vi "Begin.vi"(8 "error in":errorcluster) -> (0 "error out":errorcluster)   [LabVIEW 2020]
doc: "Called before other user functions, this VI is expected to open initial I/O refnums, load in file data, and do all program initialization. Notice that the <B>error out</B> terminal is simply used for data flow. Wiring it to other structures or subVIs ensures that this VI runs first."
uses:
  <vilib>/Rock Robotics/WPI/DriverStation/WPI_DriverStationRobotMode2.ctl
  <vilib>/Rock Robotics/WPI/Joystick/WPI_JoystickDeviceEnum.ctl
  <vilib>/Rock Robotics/WPI/Solenoid/WPI_SolenoidChannel.ctl
  <vilib>/Rock Robotics/SystemInterfaces/DIO/FPGA_DIOPWMChannel.ctl
  <vilib>/Rock Robotics/SystemInterfaces/DIO/FPGA_DIOChannel.ctl
  <vilib>/Rock Robotics/SystemInterfaces/AI/FPGA_AIChannel.ctl
  Robot Global Data.vi
  <vilib>/Rock Robotics/WPI/Solenoid/WPI_SolenoidOpenDouble.vi
  <vilib>/Rock Robotics/WPI/MotorControl/WPI_MotorControlOpen SPARK.vi
  <vilib>/Rock Robotics/WPI/Accelerometer/InternalAccelerometer/WPI_AccelerometerInternalOpen.vi
  <vilib>/Rock Robotics/WPI/SafetyOutput/WPI_SafetyOutputConfigMenu.ctl
  <vilib>/Rock Robotics/Network Tables/NT Write String Array.vi
  <vilib>/Rock Robotics/SystemInterfaces/AI/FPGA_AIGyroChannel.ctl
  <vilib>/Rock Robotics/SystemInterfaces/DIO/FPGA_DIORelayChannel.ctl
  <vilib>/Rock Robotics/WPI/Ultrasonic/WPI_SonarMB1010AnalogRefNum Registry Set.vi
  <vilib>/Rock Robotics/WPI/Ultrasonic/WPI_SonarMB1010AnalogOpen.vi
  <vilib>/Rock Robotics/WPI/Gyro/WPI_GyroAnalogOpen.vi
  <vilib>/Rock Robotics/WPI/RobotDrive/WPI_RobotDriveOpen2MotorWithVictorSPX.vi
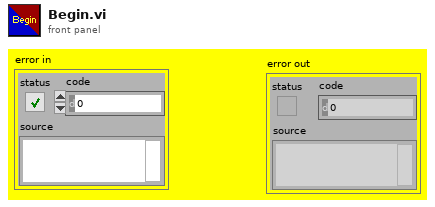
[diagram p1: front panel]
types:
  T1 = typedef "FPGA_DIOChannel.ctl" = enum8{"DIO 0", "DIO 1", "DIO 2", "DIO 3", "DIO 4", "DIO 5", "DIO 6", "DIO 7", "DIO 8", "DIO 9", "DIO MXP 0", "DIO MXP 1", "DIO MXP 2", "DIO MXP 3", "DIO MXP 4", "DIO MXP 5", "DIO MXP 6", "DIO MXP 7", "DIO MXP 8", "DIO MXP 9", "DIO MXP 10", "DIO MXP 11", "DIO MXP 12", "DIO MXP 13", "DIO MXP 14", "DIO MXP 15", "SPI Port CS1", "SPI Port CS2", "SPI Port CS3", "SPI Port MISO", "SPI Port MOSI", "Invalid"}
  T2 = enum16{"Do Nothing", "Cargo", "Low", "High", "Long Shot", "U", "Hook", "Tee"}
  T3 = typedef "FPGA_AIChannel.ctl" = enum8{"AI 0", "AI 1", "AI 2", "AI 3", "AI MXP 0", "AI MXP 1", "AI MXP 2", "AI MXP 3", "Invalid"}
  T4 = typedef "WPI_SolenoidChannel.ctl" = enum8{"Solenoid 0", "Solenoid 1", "Solenoid 2", "Solenoid 3", "Solenoid 4", "Solenoid 5", "Solenoid 6", "Solenoid 7", "Solenoid 8", "Solenoid 9", "Solenoid 10", "Solenoid 11", "Solenoid 12", "Solenoid 13", "Solenoid 14", "Solenoid 15", "Invalid"}
  T5 = typedef "FPGA_DIOPWMChannel.ctl" = enum8{"PWM 0", "PWM 1", "PWM 2", "PWM 3", "PWM 4", "PWM 5", "PWM 6", "PWM 7", "PWM 8", "PWM 9", "PWM MXP 0", "PWM MXP 1", "PWM MXP 2", "PWM MXP 3", "PWM MXP 4", "PWM MXP 5", "PWM MXP 6", "PWM MXP 7", "PWM MXP 8", "PWM MXP 9", "Invalid"}
  T6 = typedef "WPI_JoystickDeviceEnum.ctl" = enum16{"USB 0", "USB 1", "USB 2", "USB 3", "USB 4", "USB 5"}
  T7 = typedef "WPI_DriverStationRobotMode2.ctl" = enum16{"Autonomous Disabled", "Autonomous Enabled", "Teleop Disabled", "Teleop Enabled", "Disconnected", "Finish", "Test Disabled", "Test Enabled", "Emergency Stopped"}
  T8 = typedef "WPI_SafetyOutputConfigMenu.ctl" = enum16{"Enable", "Disable"}
  T9 = typedef "WPI_JoystickDevRef.ctl" = cluster{"Device":T6}
  T10 = typedef "WPI_RobotDriveDevRef.ctl" = cluster{"DevStatus":errorcluster, "Motors[]":T11[], "Square Inputs":bool, "Max Output":dbl}
  T11 = typedef "WPI_MotorControlDeviceRef.ctl" = cluster{"DeviceStatus":errorcluster, "Type":T12, "PWM":cluster{"PWM Channel":T5, "DeadBand":T13}, "CAN":cluster{"Device Number":u8, "SetOutput VI Ref":variant, "GetOutput VI Ref":variant, "Enable VI Ref":variant, "Disable VI Ref":variant, "Data":variant}, "Invert":bool, "DIO PWM":cluster{"PWM \"Enable\" Channel":T5, "DIOChannel":T1, "PWM Rate":dbl}}
  T12 = typedef "WPI_MotorControlType.ctl" = enum16{"PWM", "CAN", "DIO PWM"}
  T13 = typedef "WPI_PWMDeadband.ctl" = cluster{"Name":string, "maxPositivePwm":i32, "minPositivePwm":i32, "centerPwm":i32, "maxNegativePwm":i32, "minNegativePwm":i32, "angularRange":u16}
  T14 = typedef "FPGA_DIORelayChannel.ctl" = enum8{"Relay 0", "Relay 1", "Relay 2", "Relay 3", "Invalid"}
  T15 = typedef "WPI_RelayDevRef.ctl" = cluster{"DevStatus":errorcluster, "Relay Channel":T14, "Relay Direction":T16}
  T16 = typedef "WPI_RelayDirection.ctl" = enum16{"Both directions", "Forward only", "Reverse only"}
  T17 = typedef "WPI_DigitalOutputDevRef.ctl" = cluster{"DIO Channel":T1, "DevStatus":errorcluster}
  T18 = typedef "WPI_SolenoidDevRef.ctl" = cluster{"DevStatus":errorcluster, "Pneumatics Control Module":u8, "Forward Solenoid Channel":T4, "Reverse Solenoid Channel":T4}
  T19 = typedef "FPGA_AIGyroChannel.ctl" = enum8{"AI 0", "AI 1", "Invalid"}
  T20 = typedef "WPI_GyroDevRef.ctl" = cluster{"DevStatus":errorcluster, "Analog Channel":T3, "Gain (VoltsPerDegree/Second)":dbl, "Gyro Type":enum16{"Analog", "XRS450"}, "Handle":i32, "SPI Bus":T21, "Device Found":bool, "Sample Rate":dbl, "Calibrate On Open":bool, "Offset":dbl}
  T21 = typedef "spi_bus.ctl" = enum16{"SPI On-Board, CS0", "SPI On-Board, CS1", "SPI On-Board, CS2", "SPI On-Board, CS3", "SPI MXP", "Invalid"}
  T22 = typedef "WPI_SonarMB1010AnalogDeviceRef.ctl" = cluster{"AIDeviceRef":T23, "Scaling factor (V/in)":dbl, "Average Bits":u8}
  T23 = typedef "WPI_AnalogChannelDevRef.ctl" = cluster{"DevStatus":errorcluster, "Analog Channel":T3}
  T24 = typedef "WPI_DigitalInputDevRef.ctl" = cluster{"DevStatus":errorcluster, "DIO Channel":T1}
  T25 = typedef "WPI_AccelerometerDevRef.ctl" = cluster{"DevStatus":errorcluster, "Scaling":T26, "Analog Channels":T27, "I2C Bus":T28, "SPI Bus":T21, "Accel Range":T29, "ADXL Axes":T30, "Handle":i32, "Device Address":u8, "Accel Type":enum16{"Analog", "ADXL345 I2C", "ADXL345 SPI", "Internal", "ADXL362 SPI"}}
  T26 = typedef "WPI_AccelerometerScaling.ctl" = cluster{"Gain (VoltsPerG)":dbl, "Center Voltage":dbl}
  T27 = typedef "WPI_AccelerometerAnalogChannels.ctl" = cluster{"X-Axis":T3, "Y-Axis":T3, "Z-Axis":T3}
  T28 = typedef "i2c_bus.ctl" = enum16{"I2C On-Board", "I2C MXP", "Invalid"}
  T29 = typedef "ADXL345 Range.ctl" = u8
  T30 = typedef "WPI_AccelerometerADXL345 Axes.ctl" = cluster{"X-Axis":bool, "Y-Axis":bool, "Z-Axis":bool}
  T31 = typedef "WPI_PotentiometerDevRef.ctl" = cluster{"DevStatus":errorcluster, "Analog Channel":T3, "Invert Output":bool}
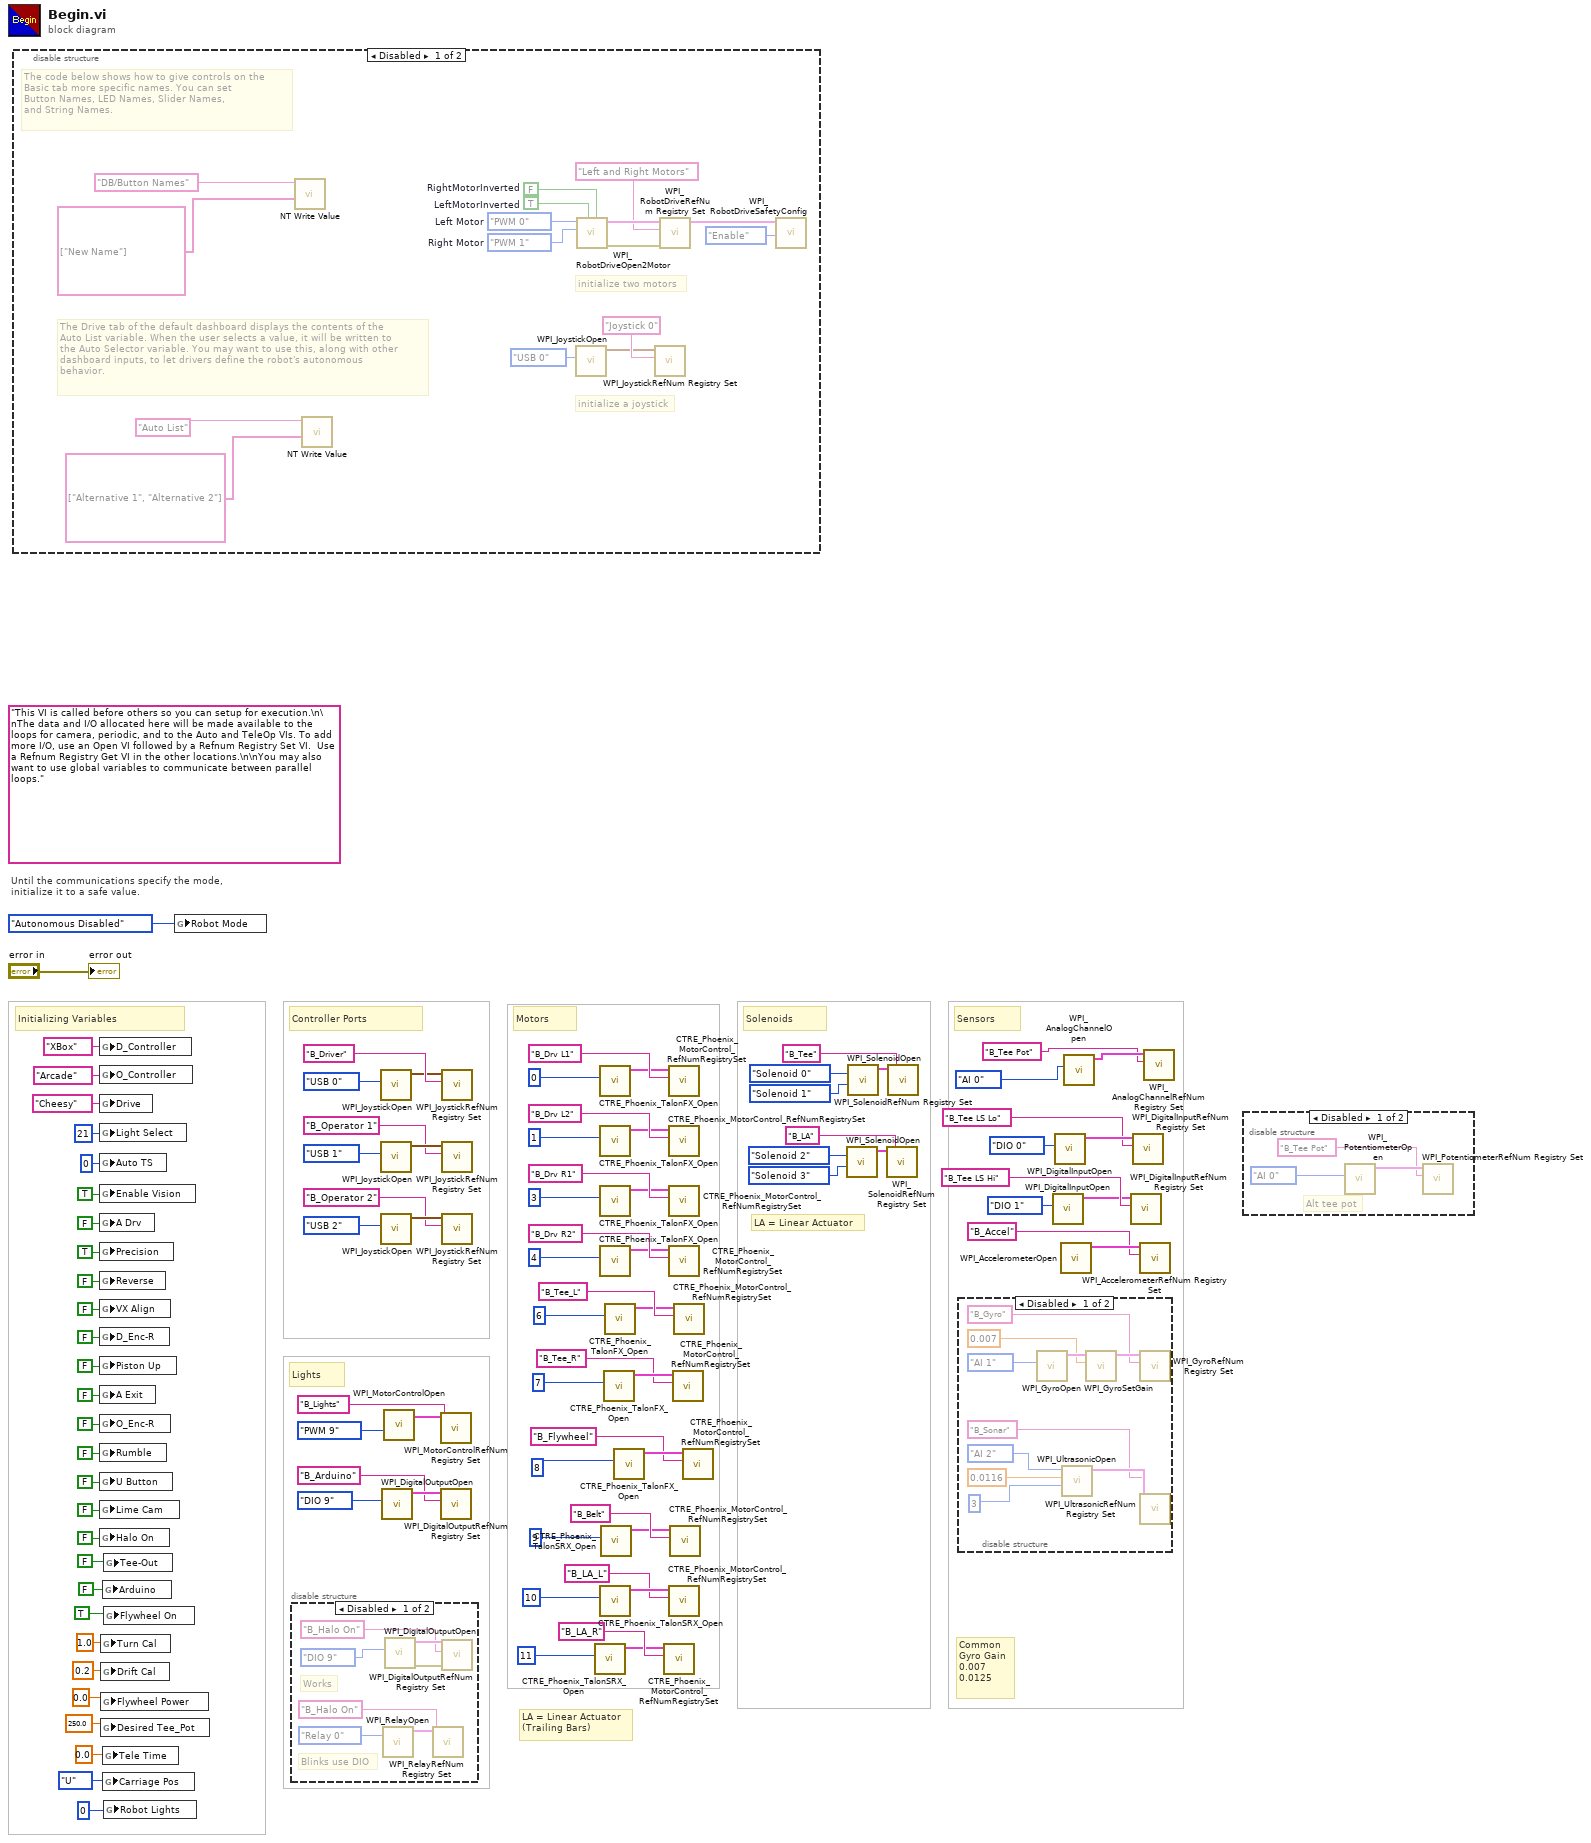
[diagram p0: block diagram]
diagram:
  (unwired) "This VI is called before others so you can setup for execution.\n\nThe data and I/O allocated here will be made available to the loops for camera, periodic, and to the Auto and TeleOp VIs. To add more I/O, use an Open VI followed by a Refnum Registry Set VI.  Use a Refnum Registry Get VI in the other locations.\n\nYou may also want to use global variables to communicate between parallel loops."
  # "LA = Linear Actuator\n(Trailing Bars)"
  # "LA = Linear Actuator"
  # "Common \nGyro Gain\n0.007\n0.0125"
  # "Sensors"
  # "Solenoids"
  # "Lights"
  # "Motors"
  # "Controller Ports"
  # "Initializing Variables"
  # "Until the communications specify the mode,\ninitialize it to a safe value."
  n1 = disable-structure shown="Disabled" {
    frame Disabled {
      w104 = FPGA_DIOPWMChannel."PWM 1"  # Right Motor
      w105 = FPGA_DIOPWMChannel."PWM 0"  # Left Motor
      w109 = TRUE  # LeftMotorInverted
      w110 = FALSE  # RightMotorInverted
      # "The Drive tab of the default dashboard displays the contents of the\nAuto List variable. When the user selects a value, it will be written to\nthe Auto Selector variable. You may want to use this, along with other\ndashboard inputs, to let drivers define the robot's autonomous\nbehavior."
      # "The code below shows how to give controls on the\nBasic tab more specific names. You can set\nButton Names, LED Names, Slider Names,\nand String Names."
      # "initialize a joystick"
      # "initialize two motors"
      n2 = call-poly <vilib>:"NT Write Value.vi"("String Array"=string[] ["New Name"], "Name"="DB/Button Names") -> ()  [unwired: 9 in, 1 out]
      n3 = call-poly <vilib>:"NT Write Value.vi"("String Array"=string[] ["Alternative 1", "Alternative 2"], "Name"="Auto List") -> ()  [unwired: 9 in, 1 out]
      n4 = call <vilib>:"WPI_JoystickOpen.vi"("JoystickDevice"=WPI_JoystickDeviceEnum."USB 0") -> ("JoystickDevRef"=w100:T9)  [unwired: 10 in]
      n5 = call-poly <vilib>:"WPI_RobotDriveOpen2Motor.vi"("Right Motor Inverted"=w110, "Left Motor Inverted"=w109, "Right Motor"=w104, "Left Motor"=w105) -> ("error out"=w106:errorcluster, "RobotDriveDevRef"=w108:T10)  [unwired: 1 in, 5 out]
      n6 = call <vilib>:"WPI_JoystickRefNum Registry Set.vi"("refnum name"="Joystick 0", "JoystickDevRef"=w100) -> ()  [unwired: 8 in, 2 out]
      n7 = call <vilib>:"WPI_RobotDriveRefNum Registry Set.vi"("error in (no error)"=w106, "refnum name"="Left and Right Motors", "RobotDriveDevRef"=w108) -> ("RobotDriveDevRef"=w103:T10)  [unwired: 1 in, 7 out]
      n8 = call <vilib>:"WPI_RobotDriveSafetyConfig.vi"("mode"=WPI_SafetyOutputConfigMenu."Enable", "RobotDriveDevRef"=w103) -> ()  [unwired: 8 in, 2 out]
    }
    frame Enabled {
    }
  }
  n9 = global write "Robot Global Data.vi" "D_Controller"("XBox" ("D_Controller")) -> ()
  n10 = global write "Robot Global Data.vi" "O_Controller"("Arcade" ("O_Controller")) -> ()
  n11 = global write "Robot Global Data.vi" "Drive"("Cheesy" ("Drive")) -> ()
  n12 = global write "Robot Global Data.vi" "Light Select"(i8 21 ("Light Select")) -> ()
  n13 = global write "Robot Global Data.vi" "Auto TS"(i8 0 ("Light Select")) -> ()
  n14 = global write "Robot Global Data.vi" "Enable Vision"(TRUE ("Enable Vision")) -> ()
  n15 = global write "Robot Global Data.vi" "A Drv"(FALSE ("Enable Vision")) -> ()
  n16 = global write "Robot Global Data.vi" "Precision"(TRUE ("Enable Vision")) -> ()
  n17 = global write "Robot Global Data.vi" "Reverse"(FALSE ("Enable Vision")) -> ()
  n18 = global write "Robot Global Data.vi" "VX Align"(FALSE ("Enable Vision")) -> ()
  n19 = global write "Robot Global Data.vi" "D_Enc-R"(FALSE ("Enable Vision")) -> ()
  n20 = global write "Robot Global Data.vi" "Piston Up"(FALSE ("Enable Vision")) -> ()
  n21 = global write "Robot Global Data.vi" "A Exit"(FALSE ("Enable Vision")) -> ()
  n22 = global write "Robot Global Data.vi" "O_Enc-R"(FALSE ("Enable Vision")) -> ()
  n23 = global write "Robot Global Data.vi" "Rumble"(FALSE ("Enable Vision")) -> ()
  n24 = global write "Robot Global Data.vi" "U Button"(FALSE ("Enable Vision")) -> ()
  n25 = global write "Robot Global Data.vi" "Lime Cam"(FALSE ("Enable Vision")) -> ()
  n26 = global write "Robot Global Data.vi" "Halo On"(FALSE ("Enable Vision")) -> ()
  n27 = global write "Robot Global Data.vi" "Turn Cal"(1.0 ("Drift Cal")) -> ()
  n28 = global write "Robot Global Data.vi" "Drift Cal"(0.2 ("Drift Cal")) -> ()
  n29 = global write "Robot Global Data.vi" "Flywheel Power"(0.0 ("Drift Cal")) -> ()
  n30 = global write "Robot Global Data.vi" "Desired Tee_Pot"(250.0 ("Drift Cal")) -> ()
  n31 = global write "Robot Global Data.vi" "Arduino"(FALSE ("Arduino")) -> ()
  n32 = global write "Robot Global Data.vi" "Tele Time"(0.0 ("Tele Time")) -> ()
  n33 = global write "Robot Global Data.vi" "Carriage Pos"(T2."U" ("Carriage Pos")) -> ()
  n34 = global write "Robot Global Data.vi" "Tee-Out"(FALSE ("Tee-Out")) -> ()
  n35 = global write "Robot Global Data.vi" "Flywheel On"(TRUE ("Flywheel On")) -> ()
  n36 = global write "Robot Global Data.vi" "Robot Lights"(i8 0 ("Robot Lights")) -> ()
  n37 = global write "Robot Global Data.vi" "Robot Mode"(WPI_DriverStationRobotMode2."Autonomous Disabled" ("Robot Mode")) -> ()
  n38 = disable-structure shown="Disabled" {
    frame Disabled {
      # "Works"
      # "Blinks use DIO"
      n39 = call <vilib>:"WPI_RelayOpen.vi"("Relay Channel"=FPGA_DIORelayChannel."Relay 0") -> ("RelayDevRef"=w117:T15)  [unwired: 9 in, 1 out]
      n40 = call <vilib>:"WPI_DigitalOutputOpen.vi"("DIO Channel"=FPGA_DIOChannel."DIO 9") -> ("error out"=w113:errorcluster, "DigitalOutputDevRef"=w114:T17)  [unwired: 9 in]
      n41 = call <vilib>:"WPI_RelayRefNum Registry Set.vi"("refnum name"="B_Halo On", "RelayDevRef"=w117) -> ()  [unwired: 8 in, 2 out]
      n42 = call <vilib>:"WPI_DigitalOutputRefNum Registry Set.vi"("error in (no error)"=w113, "refnum name"="B_Halo On", "DigitalOutputDevRef"=w114) -> ()  [unwired: 7 in, 2 out]
    }
    frame Enabled {
    }
  }
  n43 = call <vilib>:"WPI_JoystickOpen.vi"("JoystickDevice"=WPI_JoystickDeviceEnum."USB 0") -> ("JoystickDevRef"=w91:T9)  [unwired: 10 in]
  n44 = call <vilib>:"WPI_JoystickOpen.vi"("JoystickDevice"=WPI_JoystickDeviceEnum."USB 1") -> ("JoystickDevRef"=w88:T9)  [unwired: 10 in]
  n45 = call <vilib>:"WPI_JoystickOpen.vi"("JoystickDevice"=WPI_JoystickDeviceEnum."USB 2") -> ("JoystickDevRef"=w77:T9)  [unwired: 10 in]
  n46 = call <vilib>:"WPI_DigitalOutputOpen.vi"("DIO Channel"=FPGA_DIOChannel."DIO 9") -> ("DigitalOutputDevRef"=w6:T17)  [unwired: 9 in, 1 out]
  n47 = call-poly <vilib>:"WPI_MotorControlOpen.vi"("PWM Channel"=FPGA_DIOPWMChannel."PWM 9") -> ("MotorControlDeviceRef"=w65:T11)  [unwired: 9 in, 1 out]
  n48 = call <vilib>:"WPI_MotorControlRefNum Registry Set.vi"("refnum name"="B_Lights", "MotorControlDevRef"=w65) -> ()  [unwired: 8 in, 2 out]
  n49 = call <vilib>:"WPI_DigitalOutputRefNum Registry Set.vi"("refnum name"="B_Arduino", "DigitalOutputDevRef"=w6) -> ()  [unwired: 8 in, 2 out]
  n50 = call <vilib>:"WPI_JoystickRefNum Registry Set.vi"("refnum name"="B_Driver", "JoystickDevRef"=w91) -> ()  [unwired: 8 in, 2 out]
  n51 = call <vilib>:"WPI_JoystickRefNum Registry Set.vi"("refnum name"="B_Operator 1", "JoystickDevRef"=w88) -> ()  [unwired: 8 in, 2 out]
  n52 = call <vilib>:"WPI_JoystickRefNum Registry Set.vi"("refnum name"="B_Operator 2", "JoystickDevRef"=w77) -> ()  [unwired: 8 in, 2 out]
  n53 = call <vilib>:"CTRE_Phoenix_TalonSRX_Open.vi"("Device Number"=u8 11) -> ("PhoenixMotorControlDevRef"=w23:T11)  [unwired: 9 in, 1 out]
  n54 = call <vilib>:"CTRE_Phoenix_TalonFX_Open.vi"("Device Number"=u8 0) -> ("PhoenixMotorControlDevRef"=w49:T11)  [unwired: 9 in, 1 out]
  n55 = call <vilib>:"CTRE_Phoenix_TalonFX_Open.vi"("Device Number"=u8 1) -> ("PhoenixMotorControlDevRef"=w48:T11)  [unwired: 9 in, 1 out]
  n56 = call <vilib>:"CTRE_Phoenix_TalonFX_Open.vi"("Device Number"=u8 3) -> ("PhoenixMotorControlDevRef"=w47:T11)  [unwired: 9 in, 1 out]
  n57 = call <vilib>:"CTRE_Phoenix_TalonFX_Open.vi"("Device Number"=u8 4) -> ("PhoenixMotorControlDevRef"=w46:T11)  [unwired: 9 in, 1 out]
  n58 = call <vilib>:"CTRE_Phoenix_TalonSRX_Open.vi"("Device Number"=u8 10) -> ("PhoenixMotorControlDevRef"=w37:T11)  [unwired: 9 in, 1 out]
  n59 = call <vilib>:"CTRE_Phoenix_TalonSRX_Open.vi"("Device Number"=u8 9) -> ("PhoenixMotorControlDevRef"=w43:T11)  [unwired: 9 in, 1 out]
  n60 = call <vilib>:"CTRE_Phoenix_TalonFX_Open.vi"("Device Number"=u8 7) -> ("PhoenixMotorControlDevRef"=w28:T11)  [unwired: 9 in, 1 out]
  n61 = call <vilib>:"CTRE_Phoenix_TalonFX_Open.vi"("Device Number"=u8 6) -> ("PhoenixMotorControlDevRef"=w29:T11)  [unwired: 9 in, 1 out]
  n62 = call <vilib>:"CTRE_Phoenix_TalonFX_Open.vi"("Device Number"=u8 8) -> ("PhoenixMotorControlDevRef"=w34:T11)  [unwired: 9 in, 1 out]
  n63 = call <vilib>:"CTRE_Phoenix_MotorControl_RefNumRegistrySet.vi"("refnum name"="B_LA_R", "PhoenixMotorControlDevRef"=w23) -> ()  [unwired: 8 in, 2 out]
  n64 = call <vilib>:"CTRE_Phoenix_MotorControl_RefNumRegistrySet.vi"("refnum name"="B_Drv L1", "PhoenixMotorControlDevRef"=w49) -> ()  [unwired: 8 in, 2 out]
  n65 = call <vilib>:"CTRE_Phoenix_MotorControl_RefNumRegistrySet.vi"("refnum name"="B_Drv L2", "PhoenixMotorControlDevRef"=w48) -> ()  [unwired: 8 in, 2 out]
  n66 = call <vilib>:"CTRE_Phoenix_MotorControl_RefNumRegistrySet.vi"("refnum name"="B_Drv R1", "PhoenixMotorControlDevRef"=w47) -> ()  [unwired: 8 in, 2 out]
  n67 = call <vilib>:"CTRE_Phoenix_MotorControl_RefNumRegistrySet.vi"("refnum name"="B_Drv R2", "PhoenixMotorControlDevRef"=w46) -> ()  [unwired: 8 in, 2 out]
  n68 = call <vilib>:"CTRE_Phoenix_MotorControl_RefNumRegistrySet.vi"("refnum name"="B_LA_L", "PhoenixMotorControlDevRef"=w37) -> ()  [unwired: 8 in, 2 out]
  n69 = call <vilib>:"CTRE_Phoenix_MotorControl_RefNumRegistrySet.vi"("refnum name"="B_Belt", "PhoenixMotorControlDevRef"=w43) -> ()  [unwired: 8 in, 2 out]
  n70 = call <vilib>:"CTRE_Phoenix_MotorControl_RefNumRegistrySet.vi"("refnum name"="B_Tee_R", "PhoenixMotorControlDevRef"=w28) -> ()  [unwired: 8 in, 2 out]
  n71 = call <vilib>:"CTRE_Phoenix_MotorControl_RefNumRegistrySet.vi"("refnum name"="B_Tee_L", "PhoenixMotorControlDevRef"=w29) -> ()  [unwired: 8 in, 2 out]
  n72 = call <vilib>:"CTRE_Phoenix_MotorControl_RefNumRegistrySet.vi"("refnum name"="B_Flywheel", "PhoenixMotorControlDevRef"=w34) -> ()  [unwired: 8 in, 2 out]
  n73 = call-poly <vilib>:"WPI_SolenoidOpen.vi"("Reverse Solenoid Channel"=WPI_SolenoidChannel."Solenoid 3", "Forward Solenoid Channel"=WPI_SolenoidChannel."Solenoid 2") -> ("SolenoidDevRef"=w22:T18)  [unwired: 8 in, 1 out]
  n74 = call-poly <vilib>:"WPI_SolenoidOpen.vi"("Reverse Solenoid Channel"=WPI_SolenoidChannel."Solenoid 1", "Forward Solenoid Channel"=WPI_SolenoidChannel."Solenoid 0") -> ("SolenoidDevRef"=w79:T18)  [unwired: 8 in, 1 out]
  n75 = call <vilib>:"WPI_SolenoidRefNum Registry Set.vi"("refnum name"="B_LA", "SolenoidDevRef"=w22) -> ()  [unwired: 8 in, 2 out]
  n76 = call <vilib>:"WPI_SolenoidRefNum Registry Set.vi"("refnum name"="B_Tee", "SolenoidDevRef"=w79) -> ()  [unwired: 8 in, 2 out]
  n77 = disable-structure shown="Disabled" {
    frame Disabled {
      n78 = call-poly <vilib>:"WPI_GyroOpen.vi"("Analog Channel"=FPGA_AIGyroChannel."AI 1") -> ("GyroDevRef"=w126:T20)  [unwired: 8 in, 2 out]
      n79 = call-poly <vilib>:"WPI_UltrasonicOpen.vi"("Average Bits"=u8 3, "Scaling factor (V/in)"=0.0116, "Analog Channel"=FPGA_AIChannel."AI 2") -> ("SonarMB1010AnalogDevRef"=w122:T22)  [unwired: 7 in, 1 out]
      n80 = call <vilib>:"WPI_GyroSetGain.vi"("Gain (VoltsPerDegree/Second)"=0.007, "GyroDevRef"=w126) -> ("GyroDevRef"=w127:T20)  [unwired: 8 in, 1 out]
      n81 = call <vilib>:"WPI_GyroRefNum Registry Set.vi"("refnum name"="B_Gyro", "GyroDevRef"=w127) -> ()  [unwired: 8 in, 2 out]
      n82 = call-poly <vilib>:"WPI_UltrasonicRefNum Registry Set.vi"("refnum name"="B_Sonar", "SonarMB1010AnalogDevRef"=w122) -> ()  [unwired: 8 in, 2 out]
    }
    frame Enabled {
    }
  }
  n83 = call <vilib>:"WPI_DigitalInputOpen.vi"("DIO Channel"=FPGA_DIOChannel."DIO 1") -> ("DigitalInputDevRef"=w15:T24)  [unwired: 9 in, 1 out]
  n84 = call <vilib>:"WPI_DigitalInputOpen.vi"("DIO Channel"=FPGA_DIOChannel."DIO 0") -> ("DigitalInputDevRef"=w41:T24)  [unwired: 9 in, 1 out]
  n85 = call-poly <vilib>:"WPI_AccelerometerOpen.vi"() -> ("AccelerometerDevRef"=w58:T25)  [unwired: 10 in, 1 out]
  n86 = call <vilib>:"WPI_AnalogChannelOpen.vi"("Analog Channel"=FPGA_AIChannel."AI 0") -> ("AIDeviceRef"=w13:T23)  [unwired: 9 in, 1 out]
  n87 = call <vilib>:"WPI_DigitalInputRefNum Registry Set.vi"("refnum name"="B_Tee LS Hi", "DigitalInputDevRef"=w15) -> ()  [unwired: 8 in, 2 out]
  n88 = call <vilib>:"WPI_DigitalInputRefNum Registry Set.vi"("refnum name"="B_Tee LS Lo", "DigitalInputDevRef"=w41) -> ()  [unwired: 8 in, 2 out]
  n89 = call <vilib>:"WPI_AccelerometerRefNum Registry Set.vi"("refnum name"="B_Accel", "AccelerometerDevRef"=w58) -> ()  [unwired: 8 in, 2 out]
  n90 = call <vilib>:"WPI_AnalogChannelRefNum Registry Set.vi"("refnum name"="B_Tee Pot", "AIDeviceRef"=w13) -> ()  [unwired: 8 in, 2 out]
  n91 = disable-structure shown="Disabled" {
    frame Disabled {
      # "Alt tee pot"
      n92 = call <vilib>:"WPI_PotentiometerOpen.vi"("Analog Channel"=FPGA_AIChannel."AI 0") -> ("PotDevRef"=w130:T31)  [unwired: 9 in, 1 out]
      n93 = call <vilib>:"WPI_PotentiometerRefNum Registry Set.vi"("refnum name"="B_Tee Pot", "PotDevRef"=w130) -> ()  [unwired: 8 in, 2 out]
    }
    frame Enabled {
    }
  }
  "error out" <- "error in"
